vi "Test Main.vi"() -> ()   [LabVIEW 2020]
uses:
  Class/Test Class.lvclass
  Library/Test Class/Test Class.lvclass
  Typdefs/Enum Test.ctl
  Typdefs/Cluster Test.ctl
  Library/Typedefs/Cluster Test.ctl
  Library/Test Library.lvlib
  Library/Typedefs/Enum Test.ctl
  Class/Typedefs/Cluster Test.ctl
  Class/Typedefs/Enum Test.ctl
  Library/Test Class/Typedefs/Cluster Test.ctl
  Library/Test Class/Typedefs/Enum Test.ctl
panel:
  in  "Checkbox":bool
  out "Numeric":i32
  out "Library.Class.TypeDef:Enum":T1
  out "Library.Class.TypeDef:Cluster":T2
  out "Test Library.lvlib:Test Class.lvclass":refnum<class "Test Class.lvclass">
  out "Test Class.lvclass":refnum<class "Test Class.lvclass">
  out "Class.TypeDef:Enum":T3
  out "Class.TypeDef:Cluster":T4
  out "Library.TypeDef:Enum":T5
  out "Library.TypeDef:Cluster":T6
  out "TypeDef:Enum":T7
  out "TypeDef:Cluster":T8
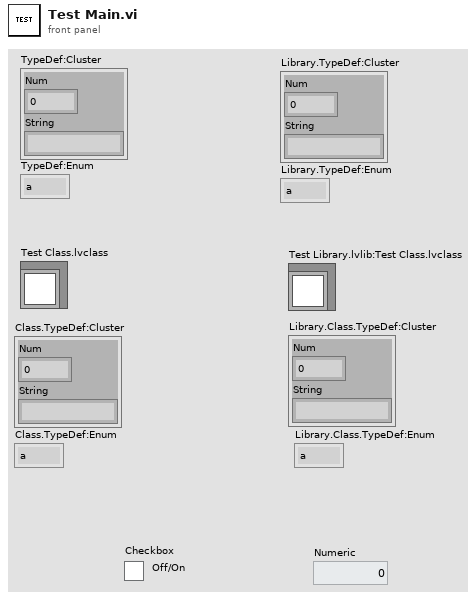
[diagram p1: front panel]
types:
  T1 = typedef "Test Library.lvlib/Test Class.lvclass/Enum Test.ctl" = enum16{"a", "b"}
  T2 = typedef "Test Library.lvlib/Test Class.lvclass/Cluster Test.ctl" = cluster{"Num":i32, "String":string}
  T3 = typedef "Test Class.lvclass/Enum Test.ctl" = enum16{"a", "b"}
  T4 = typedef "Test Class.lvclass/Cluster Test.ctl" = cluster{"Num":i32, "String":string}
  T5 = typedef "Test Library.lvlib/Enum Test.ctl" = enum16{"a", "b"}
  T6 = typedef "Test Library.lvlib/Cluster Test.ctl" = cluster{"Num":i32, "String":string}
  T7 = typedef "Enum Test.ctl" = enum16{"a", "b"}
  T8 = typedef "Cluster Test.ctl" = cluster{"Num":i32, "String":string}
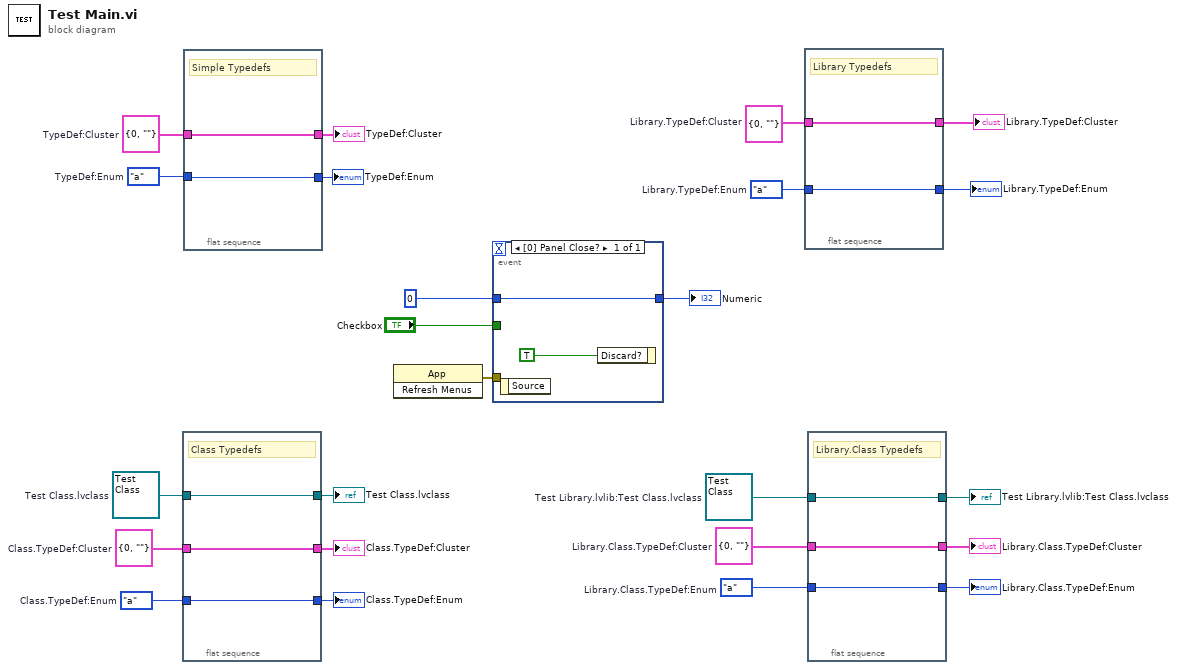
[diagram p0: block diagram]
diagram:
  w8 = refnum<class "Test Class.lvclass"> refnum  # Test Library.lvlib:Test Class.lvclass
  w4 = Enum_Test."a"  # Library.Class.TypeDef:Enum
  w6 = T2 {"Num"=0, "String"=""}  # Library.Class.TypeDef:Cluster
  w10 = refnum<class "Test Class.lvclass"> refnum  # Test Class.lvclass
  w12 = Enum_Test."a"  # Class.TypeDef:Enum
  w14 = T4 {"Num"=0, "String"=""}  # Class.TypeDef:Cluster
  w16 = Enum_Test."a"  # Library.TypeDef:Enum
  w18 = T6 {"Num"=0, "String"=""}  # Library.TypeDef:Cluster
  w22 = T8 {"Num"=0, "String"=""}  # TypeDef:Cluster
  w20 = Enum_Test."a"  # TypeDef:Enum
  n1 = flat-sequence {
    tunnel: [w27] -> w15
    tunnel: w14 -> [w27]
    tunnel: [w26] -> w13
    tunnel: w12 -> [w26]
    tunnel: [w25] -> w11
    tunnel: w10 -> [w25]
    frame #0 {
      # "Class Typedefs"
    }
  }
  n2 = flat-sequence {
    tunnel: [w29] -> w23
    tunnel: w22 -> [w29]
    tunnel: [w28] -> w21
    tunnel: w20 -> [w28]
    frame #0 {
      # "Simple Typedefs"
    }
  }
  n3 = invoke class="App" method="Refresh Menus"() -> (error out=w24:errorcluster)  [unwired: 3 in, 2 out]
  n4 = event shown="[0] Panel Close?" {
    selector: _ -> [_]
    dyn-events: _ -> [_]
    timeout: _ -> [_]
    tunnel: w24 -> [_]
    tunnel: [w30] -> w3
    tunnel: 0 -> [w30]
    tunnel: "Checkbox" -> [_]
    event Panel Close? {
      n5 = event-data() -> ()  [unwired: 1 in, 1 out]
      n6 = event-data("Discard?"=TRUE) -> ()  [unwired: 1 in, 1 out]
    }
  }
  "Numeric" <- w3
  n7 = flat-sequence {
    tunnel: [w33] -> w19
    tunnel: w18 -> [w33]
    tunnel: [w32] -> w17
    tunnel: w16 -> [w32]
    frame #0 {
      # "Library Typedefs"
    }
  }
  n8 = flat-sequence {
    tunnel: [w36] -> w9
    tunnel: w8 -> [w36]
    tunnel: [w35] -> w7
    tunnel: w6 -> [w35]
    tunnel: [w34] -> w5
    tunnel: w4 -> [w34]
    frame #0 {
      # "Library.Class Typedefs"
    }
  }
  "TypeDef:Cluster" <- w23
  "TypeDef:Enum" <- w21
  "Library.TypeDef:Cluster" <- w19
  "Library.TypeDef:Enum" <- w17
  "Class.TypeDef:Cluster" <- w15
  "Class.TypeDef:Enum" <- w13
  "Test Class.lvclass" <- w11
  "Test Library.lvlib:Test Class.lvclass" <- w9
  "Library.Class.TypeDef:Cluster" <- w7
  "Library.Class.TypeDef:Enum" <- w5
